vi "SetAddress.vi"(8 "error in (no error)":errorcluster, 9 "Address(New)":sgl, 10 "Address(Current)":u8, 11 "VISA resource name":refnum<visa-resource-name>) -> (0 "error out":errorcluster, 1 "Raw Response":string, 3 "VISA resource name out":refnum<visa-resource-name>)   [LabVIEW 2020, in "driver_flodx_pressure.lvlib"]
doc: "Must be in CONFIG mode."
uses:
  <instrlib>/RxnRover/FloDx Pressure Driver/driver_flodx_pressure.lvlib
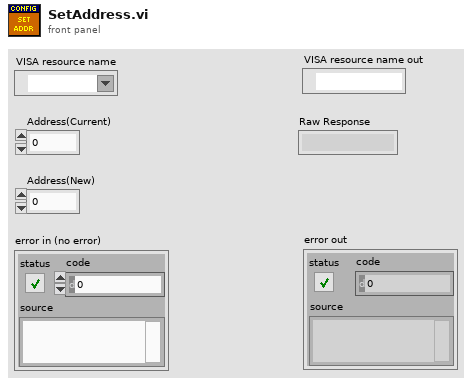
[diagram p1: front panel]
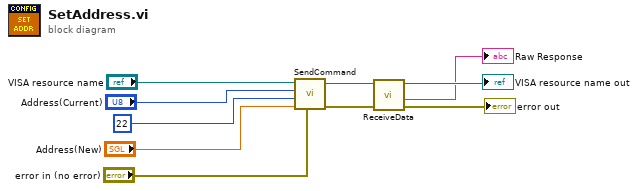
[diagram p0: block diagram]
diagram:
  n1 = call <instrlib>:"SendCommand.vi"("error in"="error in (no error)", "Parameter"="Address(New)", "Command"=u8 22, "Address"="Address(Current)", "VISA resource name"="VISA resource name") -> ("error out"=w5:errorcluster, "VISA resource name out"=w1:refnum<visa-resource-name>)  [unwired: 4 in, 1 out]
  n2 = call <instrlib>:"ReceiveData.vi"("error in (no error)"=w5, "VISA resource name"=w1) -> ("error out"=→"error out":errorcluster, "Raw Response"=→"Raw Response":string, "VISA resource name out"=→"VISA resource name out":refnum<visa-resource-name>)  [unwired: 5 in, 2 out]
